vi "write_channel_attributes.vi"(8 "error in (no error)":errorcluster, 9 "ch_number":i32, 10 "Hydraharp Settings.CH 0":T2 {"ch_offs" min=-99999 max=99999 step=1; "ch_ZeroX" min=0 max=20 step=1; "ch_level" min=0 max=800 step=10}, 11 "HDF5 Ref":T1) -> (0 "error out":errorcluster, 3 "HDF5 Ref out":T1)   [LabVIEW 2015, in "hdf5_photon_record_log.lvclass"]
uses:
  hdf5_photon_record_log.lvclass
  hydraharp_panel/hpanel_channel_settings.ctl
  <vilib>/UPVI/lvhdf5/library.llb/HDF5 Ref.ctl
  <vilib>/UPVI/lvhdf5/attribute.llb/Write Multiple Attributes.vi
  <vilib>/UPVI/lvhdf5/attribute.llb/LVH5A Operation.ctl
  <vilib>/UPVI/lvhdf5/attribute.llb/LVH5 Write Attributes.xnode
  <vilib>/Utility/VariantDataType/GetClusterInfo.vi
  <vilib>/Utility/VariantDataType/VariantType.lvlib
  <vilib>/Utility/VariantDataType/GetTypeInfo.vi
  <vilib>/UPVI/lvhdf5/attribute.llb/Cluster to Attribute Array.xnode
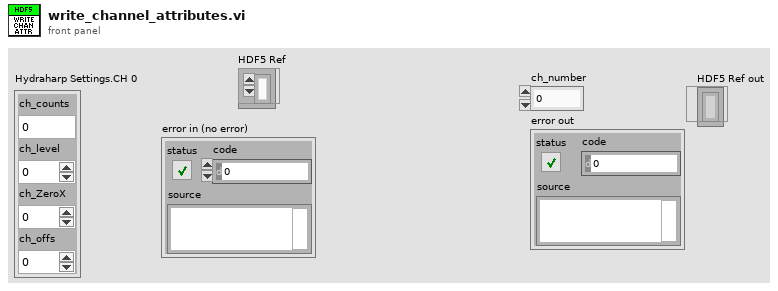
[diagram p1: front panel]
types:
  T1 = typedef "HDF5 Ref.ctl" = refnum<k1>
  T2 = typedef "hpanel_channel_settings.ctl" = cluster{"ch_counts":i32, "ch_level":i32, "ch_ZeroX":i32, "ch_offs":i32}
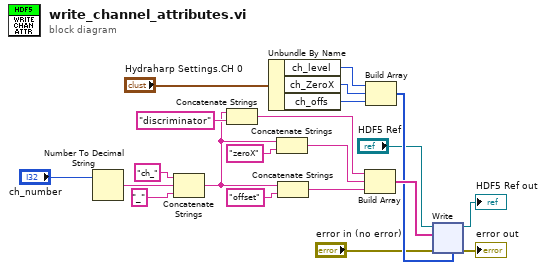
[diagram p0: block diagram]
diagram:
  n1 = Number To Decimal String(number="ch_number") -> (decimal integer string=w19:string)  [unwired: 1 in]
  n2 = Concatenate Strings("ch_" ("string"), w19, "_" ("string")) -> (w14:string)
  n3 = Concatenate Strings(w14, "discriminator" ("string")) -> (w13:string)
  n4 = Unbundle By Name("Hydraharp Settings.CH 0") -> ("ch_level"=w9:i32, "ch_ZeroX"=w8:i32, "ch_offs"=w7:i32)
  n5 = Concatenate Strings(w14, "zeroX" ("string")) -> (w12:string)
  n6 = Concatenate Strings(w14, "offset" ("string")) -> (w11:string)
  n7 = Build Array(w13, w12, w11) -> (w10:string[])
  n8 = Build Array(w9, w8, w7) -> (w6:i32[])
  n9 = xnode "Write"("HDF5 Ref"="HDF5 Ref", "error in (no error)"="error in (no error)", "Name(s)"=w10, "Value(s)"=w6) -> ("HDF5 Ref out"=→"HDF5 Ref out":T1, "error out"=→"error out":errorcluster)  [unwired: 1 in]
